vi "calculate histogram.vi"(6 "channel no.":i32, 7 "Image Ctrl Ref (as generic class)":refnum<vi>, 8 "Image Array":i16[][](array[numeric]), 9 "T for reso F for galvo":bool, 11 "Image":T1) -> ()   [LabVIEW 2017]
doc: "SciScan 1.2 160622"
uses:
  <vilib>/vision/Image Controls.llb/IMAQ Image.ctl
  Custom Controls/display palette control.ctl
  GFG/GFGfpRefGet.vi
  GFG/GFGbooleanGet.vi
  <vilib>/vision/NI_Vision_Development_Module.lvlib
  GFG/GFG library.lvlib
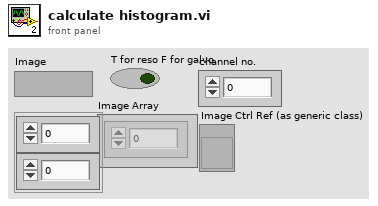
[diagram p1: front panel]
types:
  T1 = typedef "IMAQ Image.ctl" = refnum<image>
  T2 = typedef "display palette control.ctl" = enum16{"standard", "high clipping red", "low clipping blue", "high and low clipping", "high / low (full range)"}
  T3 = cluster{"WaveformChartRef":refnum<vi>, "DigitalRef":refnum<vi>, "ArrayRef":refnum<vi>, "TabControlRef":refnum<vi>, "EnumRef":refnum<vi>, "RingRef":refnum<vi>, "BooleanRef":refnum<vi>, "KnobRef":refnum<vi>, "SlideRef":refnum<vi>, "PathRef":refnum<vi>, "StringRef":refnum<vi>, "ComboBox":refnum<vi>, "WaveformGraphRef":refnum<vi>}
  T4 = cluster{"Conversion Method":u32, "Minimum Value":i32, "Maximum Value":i32, "Number Of Shifts":i32}
  T5 = cluster{"Histogram Graph":cluster{"Starting Value":sgl, "Incremental Value":sgl, "Histogram":u32[]}, i32, i32}
  T6 = cluster{"Starting Value":sgl, "Incremental Value":sgl, "Histogram":u32[]}
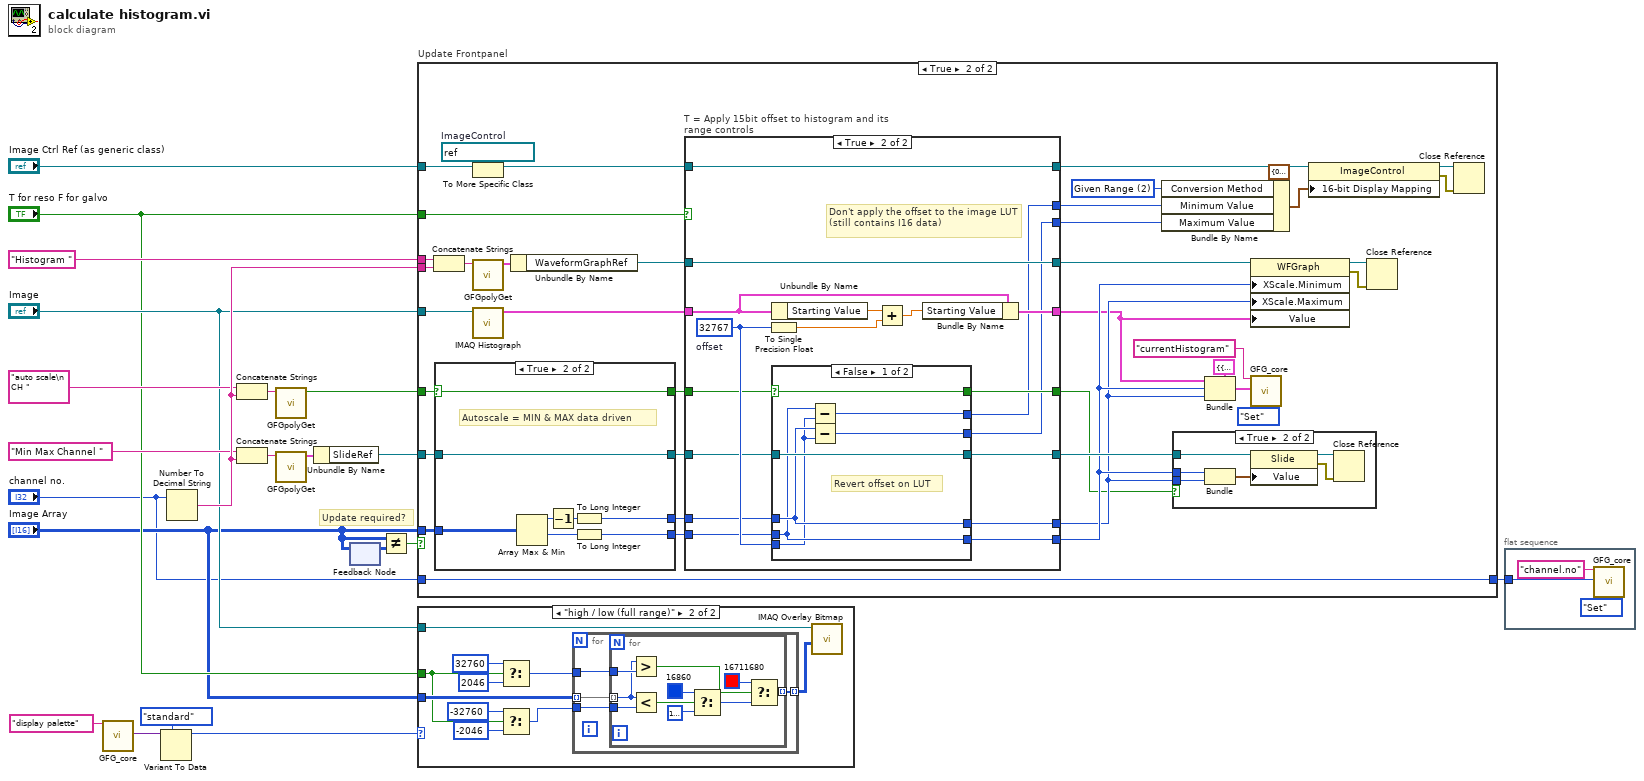
[diagram p0: block diagram]
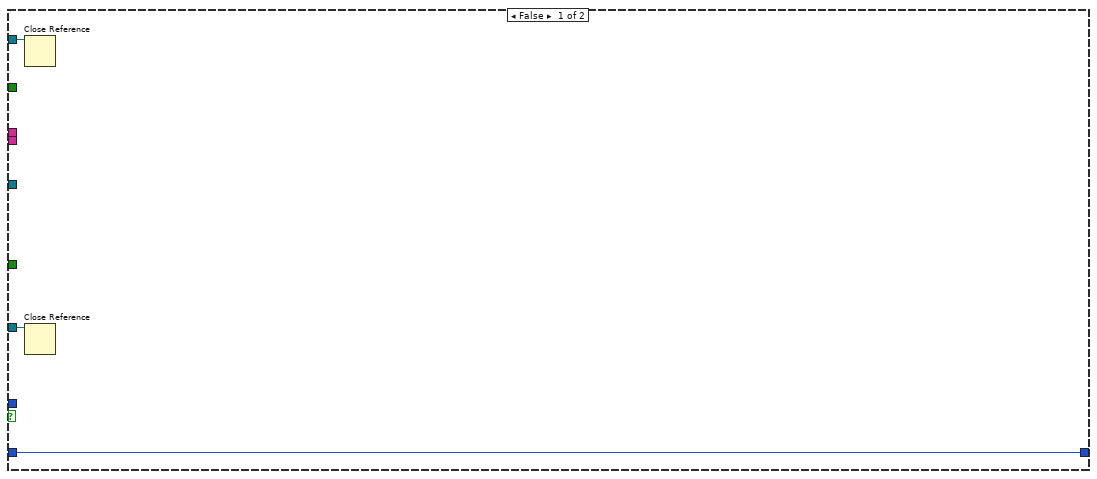
[diagram p2: hidden frame]
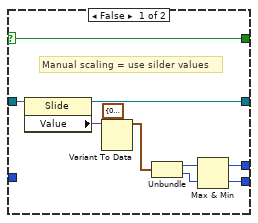
[diagram p4: hidden frame]
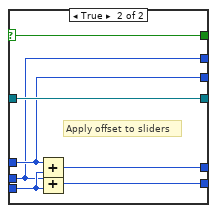
[diagram p6: hidden frame]
diagram:
  # "Update required?"
  n1 = call "GFG_core.vi"("Variable Name in"="display palette") -> ("Variant Out"=w11:variant)  [unwired: 12 in, 6 out]
  n2 = Variant To Data(type=display_palette_control."standard" ("display palette"), Variant=w11) -> (data=w10:T2)  [unwired: 1 in, 1 out]
  n3 = Number To Decimal String(number="channel no.") -> (decimal integer string=w20:string)  [unwired: 1 in]
  n4 = Concatenate Strings("auto scale\n      CH " ("Variable Name in"), w20) -> (w17:string)
  n5 = Concatenate Strings("Min Max Channel " ("Variable Name in"), w20) -> (w21:string)
  n6 = call-poly "GFGpolyGet.vi"("Variable Name in"=w17) -> ("Boolean Value OUT"=w7:bool)  [unwired: 9 in, 1 out]
  n7 = call-poly "GFGpolyGet.vi"("Variable Name in"=w21) -> ("output cluster"=w18:T3)  [unwired: 9 in, 1 out]
  n8 = Unbundle By Name(w18) -> ("SlideRef"=w1:refnum<vi>)
  n9 = feedback #1() -> (w3:i16[][])  [unwired: 1 in]
  n10 = feedback-in #1("Image Array") -> ()
  n11 = Not Equal?(x="Image Array", y=w3) -> (x != y?=w2:bool)
  n12 = case "Update Frontpanel" shown="True" w2 {
    tunnel: w20 -> [_ w63]
    tunnel: "Histogram " ("string") -> [_ w62]
    tunnel: "Image Ctrl Ref (as generic class)" -> [w24 w60]
    tunnel: "Image" -> [_ w58]
    tunnel: "T for reso F for galvo" -> [_ w49]
    tunnel: w7 -> [_ w34]
    tunnel: "Image Array" -> [_ w39]
    tunnel: w1 -> [w23 w33]
    tunnel: "channel no." -> [w22 w38]
    tunnel: [w22 w38] -> w4
    frame False {
      n13 = Close Reference(reference=w24) -> ()  [unwired: 1 in, 1 out]
      n14 = Close Reference(reference=w23) -> ()  [unwired: 1 in, 1 out]
    }
    frame True {
      w59 = refnum<vi> refnum  # ImageControl
      w26 = u32 2 items=["Full Dynamic", "Downshift", "Given Range", "90% Dynamic", "Given Percent Range"] ("16-bit Display Mapping:Conversion Method")
      n15 = Concatenate Strings(w62, w63) -> (w61:string)
      n16 = case shown="True" w34 {
        selector: w34 -> [w73 w80]
        tunnel: w39 -> [_ w87]
        tunnel: [w75 w86] -> w36
        tunnel: [w74 w85] -> w35
        tunnel: w33 -> [w72 w81]
        tunnel: [w71 w81] -> w32
        tunnel: [w73 w80] -> w31
        frame False {
          # "Manual scaling = use silder values"
          n17 = property class="Slide"(reference=w72) -> (reference out=w71:refnum<vi>, "Value"=w70:variant)  [unwired: 1 in, 1 out]
          n18 = Variant To Data(type=cluster{i32, i32} {0, 2048} ("channel1"), Variant=w70) -> (data=w76:cluster{i32, i32})  [unwired: 1 in, 1 out]
          n19 = Unbundle(w76) -> (w77:i32, w78:i32)
          n20 = Max & Min(x=w77, y=w78) -> (max(x,y)=w75:i32, min(x,y)=w74:i32)
        }
        frame True {
          # "Autoscale = MIN & MAX data driven"
          n21 = Array Max & Min(array=w87) -> (max value=w84:i16, min value=w82:i16)  [unwired: 2 out]
          n22 = Decrement(x=w84) -> (x-1=w83:i16)
          n23 = To Long Integer(number=w83) -> (32bit integer=w86:i32)
          n24 = To Long Integer(number=w82) -> (32bit integer=w85:i32)
        }
      }
      n25 = To More Specific Class(target class=w59, reference=w60) -> (specific class reference=w43:refnum<vi>)  [unwired: 1 in, 1 out]
      n26 = call-poly "GFGpolyGet.vi"("Variable Name in"=w61) -> ("output cluster"=w46:T3)  [unwired: 9 in, 1 out]
      n27 = call "IMAQ Histograph"("Image"=w58) -> ("Histogram Graph"=w48:T6)  [unwired: 7 in, 3 out]
      n28 = Unbundle By Name(w46) -> ("WaveformGraphRef"=w45:refnum<vi>)
      n29 = case "T = Apply 15bit offset to histogram and its range controls" shown="True" w49 {
        tunnel: w36 -> [w91 w104]
        tunnel: w35 -> [w90 w103]
        tunnel: [w91 w112] -> w40
        tunnel: [w90 w111] -> w41
        tunnel: [w91 w95] -> w27
        tunnel: [w90 w96] -> w28
        tunnel: w48 -> [w94 w108]
        tunnel: [w94 w105] -> w37
        tunnel: [w93 w101] -> w47
        tunnel: w45 -> [w93 w101]
        tunnel: w32 -> [w92 w98]
        tunnel: [w92 w97] -> w44
        tunnel: w43 -> [w89 w102]
        tunnel: [w89 w102] -> w42
        tunnel: w31 -> [w88 w100]
        tunnel: [w88 w99] -> w30
        frame False {
        }
        frame True {
          w107 = 32767  # offset
          # "Don't apply the offset to the image LUT (still contains I16 data)"
          n30 = To Single Precision Float(number=w107) -> (single precision float=w106:sgl)
          n31 = Unbundle By Name(w108) -> ("Starting Value"=w109:sgl)
          n32 = case shown="False" w100 {
            selector: w100 -> [w119 w123]
            tunnel: [w117 w126] -> w112
            tunnel: [w115 w125] -> w111
            tunnel: w107 -> [w114 w124]
            tunnel: w104 -> [w117 w121]
            tunnel: w103 -> [w115 w120]
            tunnel: [w119 w123] -> w99
            tunnel: w98 -> [w118 w122]
            tunnel: [w118 w122] -> w97
            tunnel: [w116 w121] -> w95
            tunnel: [w113 w120] -> w96
            frame False {
              # "Revert offset on LUT"
              n33 = Subtract(x=w115, y=w114) -> (x-y=w113:i32)
              n34 = Subtract(x=w117, y=w114) -> (x-y=w116:i32)
            }
            frame True {
              # "Apply offset to sliders"
              n35 = Add(x=w121, y=w124) -> (x+y=w126:i32)
              n36 = Add(x=w120, y=w124) -> (x+y=w125:i32)
            }
          }
          n37 = Add(x=w109, y=w106) -> (x+y=w110:sgl)
          n38 = Bundle By Name(cluster=w108, "Starting Value"=w110) -> (w105:T6)
        }
      }
      n39 = Bundle By Name(cluster=T4 {"Conversion Method"=0, "Minimum Value"=0, "Maximum Value"=0, "Number Of Shifts"=0} ("16-bit Display Mapping:All Elements"), "Conversion Method"=w26, "Minimum Value"=w28, "Maximum Value"=w27) -> (w25:T4)
      n40 = case shown="True" w30 {
        tunnel: w44 -> [_ w66]
        tunnel: w41 -> [_ w65]
        tunnel: w40 -> [_ w64]
        frame False {
          # "No need to be set"
        }
        frame True {
          n41 = Bundle(w65, w64) -> (w69:cluster{i32, i32})  [unwired: 1 in]
          n42 = property class="Slide"(reference=w66, "Value"=w69) -> (reference out=w68:refnum<vi>, error out=w67:errorcluster)  [unwired: 1 in]
          n43 = Close Reference(reference=w68, error in (no error)=w67) -> ()  [unwired: 1 out]
        }
      }
      n44 = Bundle(cluster=T5 {"Histogram Graph"={"Starting Value"=0.0, "Incremental Value"=0.0, "Histogram"=[]}, 0, 0}, "Histogram Graph"=w37, w41, w40) -> (w51:T5)
      n45 = property class="WFGraph"(reference=w47, "XScale.Minimum"=w41, "XScale.Maximum"=w40, "Value"=w37) -> (reference out=w54:refnum<vi>, error out=w55:errorcluster)  [unwired: 1 in]
      n46 = call "GFG_core.vi"("Variable Name in"="currentHistogram", "Variant in"=w51, "Action"=enum16{"Init", "Set", "Get", "Clear"}."Set") -> ()  [unwired: 10 in, 7 out]
      n47 = property class="ImageControl"(reference=w42, "16-bit Display Mapping"=w25) -> (reference out=w52:refnum<vi>, error out=w53:errorcluster)  [unwired: 1 in]
      n48 = Close Reference(reference=w54, error in (no error)=w55) -> ()  [unwired: 1 out]
      n49 = Close Reference(reference=w52, error in (no error)=w53) -> ()  [unwired: 1 out]
    }
  }
  n50 = case shown="\"high / low (full range)\"" w10 {
    tunnel: "Image" -> [_ w136]
    tunnel: "Image Array" -> [_ w135]
    tunnel: "T for reso F for galvo" -> [_ w127]
    frame Default {
    }
    frame "high / low (full range)" {
      n51 = Select(t=i16 32760 ("n"), s=w127, f=i16 2046 ("n")) -> (s? t:f=w128:i16)
      n52 = Select(t=i16 -32760 ("n"), s=w127, f=i16 -2046 ("n")) -> (s? t:f=w129:i16)
      n53 = for {
        tunnel: w135 -> [w140] mode=indexing
        tunnel: w128 -> [w139]
        tunnel: [w138] -> w134 mode=indexing
        tunnel: w129 -> [w137]
        n54 = for {
          tunnel: w140 -> [w146] mode=indexing
          tunnel: w139 -> [w150]
          tunnel: [w147] -> w138 mode=indexing
          tunnel: w137 -> [w145]
          n55 = Greater?(x=w146, y=w150) -> (0:w149:bool)
          n56 = Less?(x=w146, y=w145) -> (x < y?=w144:bool)
          n57 = Select(t=u32 16860, s=w144, f=u32 16777216) -> (s? t:f=w142:u32)
          n58 = Select(t=u32 16711680, s=w149, f=w142) -> (s? t:f=w147:u32)
        }
      }
      n59 = call "IMAQ Overlay Bitmap"("Bitmap"=w134, "Image"=w136) -> ()  [unwired: 8 in, 2 out]
    }
  }
  n60 = flat-sequence {
    tunnel: w4 -> [w152]
    frame #0 {
      n61 = call "GFG_core.vi"("Variable Name in"="channel.no", "Variant in"=w152, "Action"=enum16{"Init", "Set", "Get", "Clear"}."Set") -> ()  [unwired: 10 in, 7 out]
    }
  }
